vi "Config IQ Calibration.vi"(0 "VISA Resource Name":refnum<visa-resource-name>, 1 "Frequency Start (0.1)":dbl=0.1 format="%.5f", 3 "Frequency Stop (1000.00)":dbl=1000.0 format="%.5f", 5 "Calibration Type (0:User)":u16(ring) items=["User", "Revert to Default", "Full"], 11 "error in (no error)":errorcluster {"code" format="%.0x"}) -> (4 "VISA Resource Name Out":refnum<visa-resource-name>, 15 "error out":errorcluster {"code" format="%.0x"})   [LabVIEW 2012, in "Agilent ESG Series.lvlib"]
doc: "This VI is used to set the controls and the parameters associated with instrument calibration."
uses:
  <instrlib>/Agilent ESG Series/Agilent ESG Series.lvlib
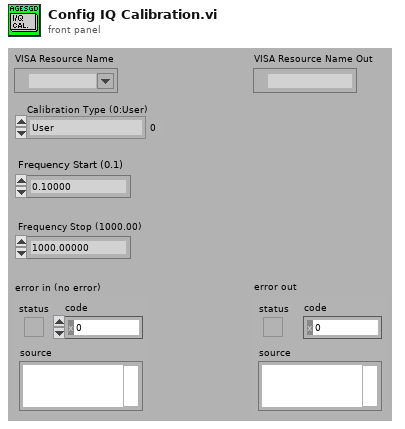
[diagram p1: front panel]
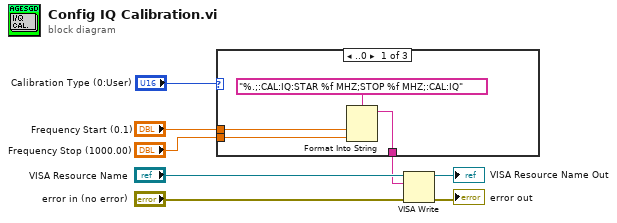
[diagram p0: block diagram]
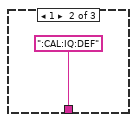
[diagram p2: hidden frame]
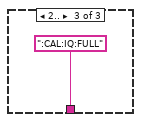
[diagram p3: hidden frame]
diagram:
  n1 = case shown="..0" "Calibration Type (0:User)" {
    tunnel: [w11 ":CAL:IQ:DEF" ":CAL:IQ:FULL"] -> w4
    tunnel: "Frequency Start (0.1)" -> [w10 _ _]
    tunnel: "Frequency Stop (1000.00)" -> [w9 _ _]
    frame ..0 {
      n2 = Format Into String(format string="%.;:CAL:IQ:STAR %f MHZ;STOP %f MHZ;:CAL:IQ", w10, w9) -> (resulting string=w11:string)  [unwired: 2 in, 1 out]
    }
    frame 1 {
    }
    frame 2.. {
    }
  }
  n3 = VISA Write(VISA resource name="VISA Resource Name", write buffer=w4, error in (no error)="error in (no error)") -> (VISA resource name out=→"VISA Resource Name Out":refnum<visa-resource-name>, error out=→"error out":errorcluster)  [unwired: 1 out]
